vi "RFH-read-common_format.vi"(7 "file path (dialog if empty)":path, 8 "error in":errorcluster) -> (0 "error out":errorcluster, 2 "Common Format":T1)   [LabVIEW 2020, in "RFH-Reflection_File_Handler.lvlib"]
uses:
  RFH-Reflection_File_Handler.lvlib
  RFH-common_data_format.ctl
panel:
  out "string array 2":string[][](array[string])
  out "string array":string[](array[string])
  out "after substring":string
  out "text":string
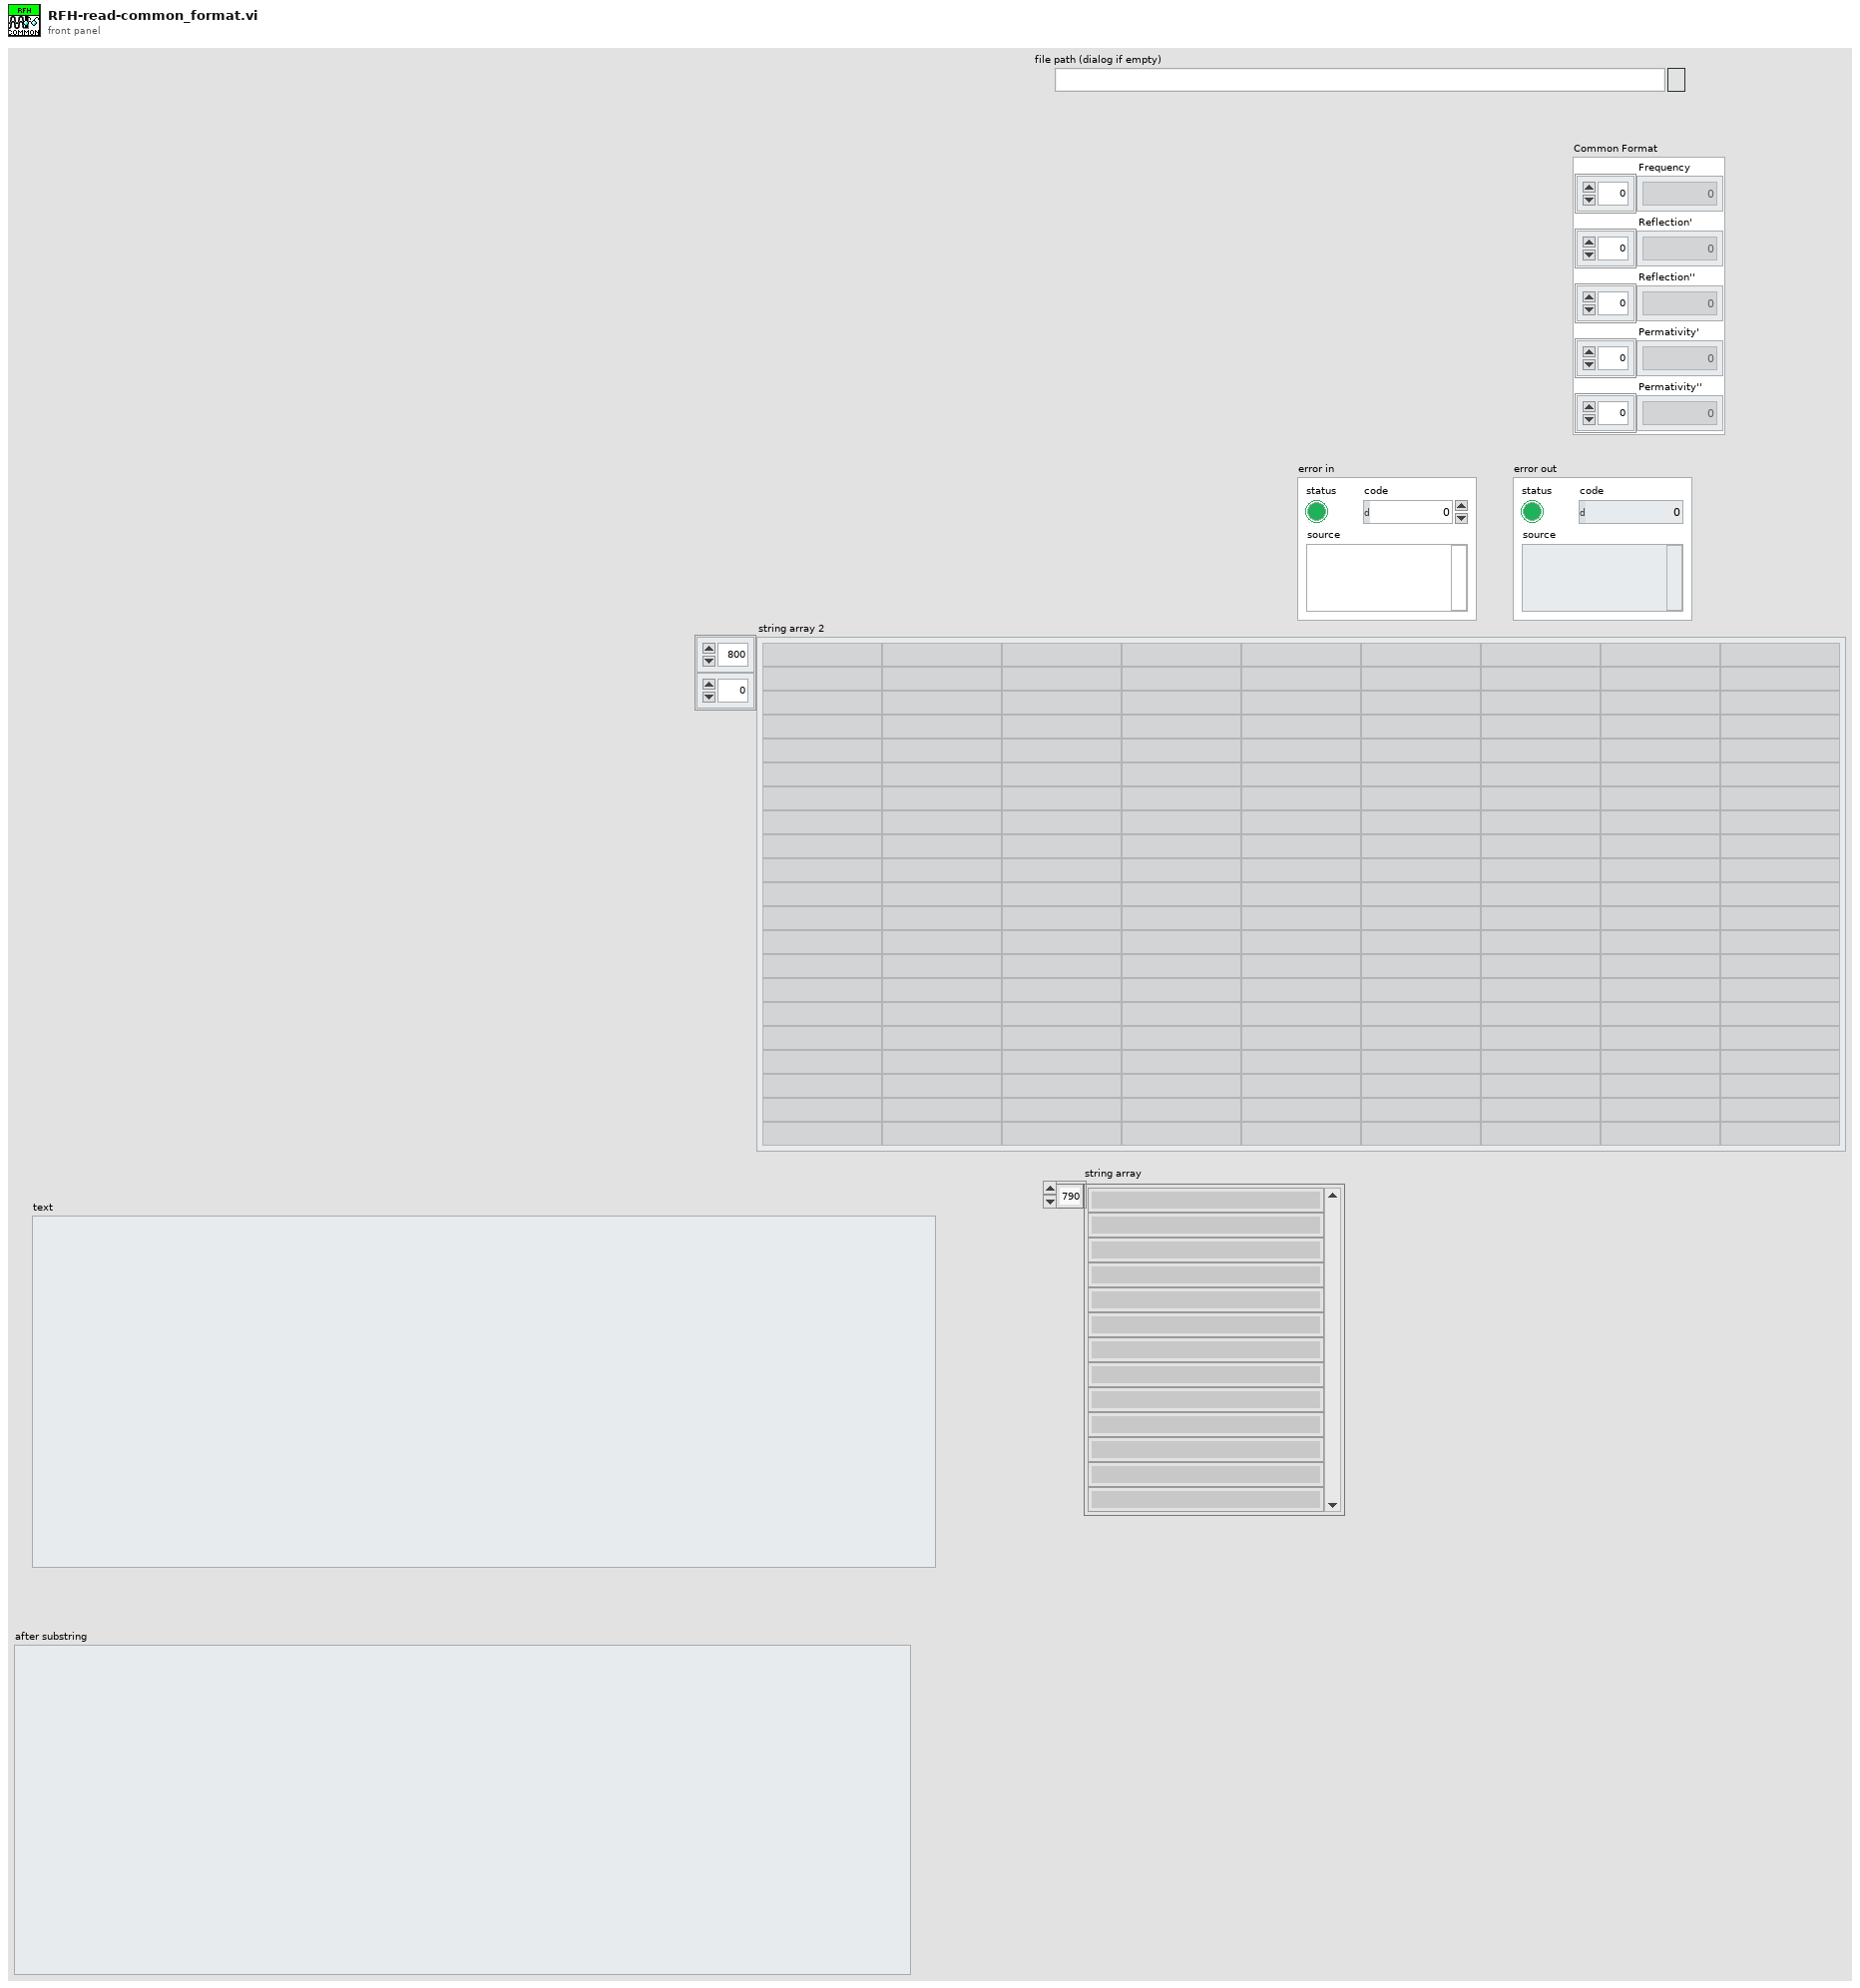
[diagram p1: front panel]
types:
  T1 = typedef "RFH-Reflection_File_Handler.lvlib/RFH-common_data_format.ctl" = cluster{"Frequency":dbl[], "Reflection'":dbl[], "Reflection''":dbl[], "Permativity'":dbl[], "Permativity''":dbl[]}
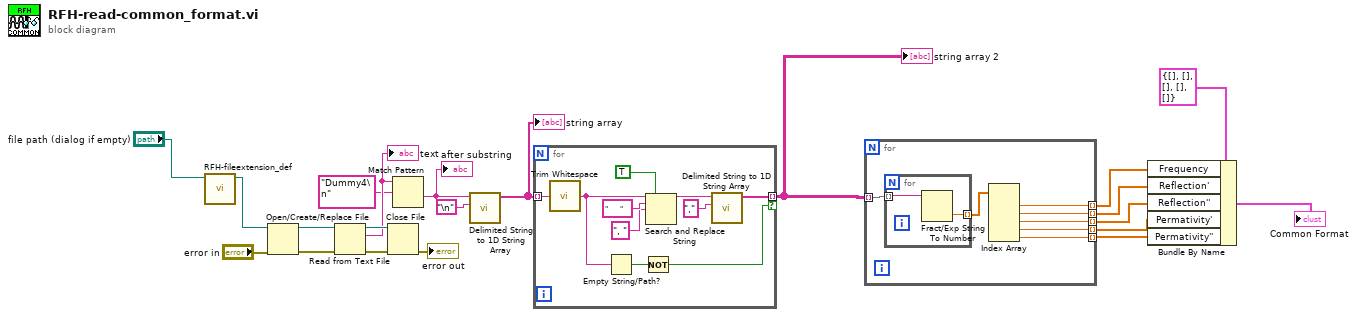
[diagram p0: block diagram]
diagram:
  n1 = call "RFH-fileextension_def.vi"("Path in"="file path (dialog if empty)") -> ("Path with file extention"=w1:path)  [unwired: 9 in, 1 out]
  n2 = Open/Create/Replace File(file path (use dialog)=w1, error in="error in") -> (refnum out=w21:refnum<file>, error out=w18:errorcluster)  [unwired: 4 in, 1 out]
  n3 = Read from Text File(file (use dialog)=w21, error in=w18) -> (refnum out=w20:refnum<file>, text=w17:string, error out=w19:errorcluster)  [unwired: 2 in, 1 out]
  "text" <- w17
  n4 = Close File(refnum=w20, error in=w19) -> (error out=→"error out":errorcluster)  [unwired: 1 out]
  n5 = Match Pattern(string=w17, regular expression="Dummy4\n" ("search string/char (-)")) -> (after substring=w13:string)  [unwired: 1 in, 3 out]
  "after substring" <- w13
  n6 = call <vilib>:"Delimited String to 1D String Array.vi"("delimiter"="\n", "delimited string"=w13) -> ("string array"=w14:string[])  [unwired: 9 in]
  "string array" <- w14
  n7 = for {
    tunnel: w14 -> [w31] mode=indexing
    tunnel: [w30] -> w12 mode=indexing if=w22
    n8 = call <vilib>:"Trim Whitespace.vi"("string"=w31) -> ("trimmed string"=w24:string)  [unwired: 1 in]
    n9 = Empty String/Path?(string/path=w24) -> (empty?=w23:bool)
    n10 = Not(x=w23) -> (.not. x?=w22:bool)
    n11 = Search and Replace String(replace all?=TRUE ("replace all? (F)"), input string=w24, search string="      ", replace string=", " ("replace string (\"\")")) -> (result string=w25:string)  [unwired: 4 in, 3 out]
    n12 = call <vilib>:"Delimited String to 1D String Array.vi"("delimiter"=",", "delimited string"=w25) -> ("string array"=w30:string[])  [unwired: 9 in]
  }
  "string array 2" <- w12
  n13 = for {
    tunnel: w12 -> [w38] mode=indexing
    tunnel: [w36] -> w11 mode=indexing
    tunnel: [w35] -> w10 mode=indexing
    tunnel: [w34] -> w9 mode=indexing
    tunnel: [w33] -> w8 mode=indexing
    tunnel: [w32] -> w7 mode=indexing
    n14 = for {
      tunnel: w38 -> [w40] mode=indexing
      tunnel: [w39] -> w37 mode=indexing
      n15 = Fract/Exp String To Number(string=w40) -> (number=w39:dbl)  [unwired: 3 in, 1 out]
    }
    n16 = Index Array(array=w37) -> (element #1=w36:dbl, element #2=w35:dbl, element #3=w34:dbl, element #4=w33:dbl, element #5=w32:dbl)  [unwired: 5 in]
  }
  n17 = Bundle By Name(cluster=T1 {"Frequency"=[], "Reflection'"=[], "Reflection''"=[], "Permativity'"=[], "Permativity''"=[]} ("Common Format"), "Frequency"=w11, "Reflection'"=w10, "Reflection''"=w9, "Permativity'"=w8, "Permativity''"=w7) -> (→"Common Format":T1)
